vi "例10.7  保存单幅图像.vi"() -> ()   [LabVIEW 2017]
panel:
  out "Image Out":T1(plugin-control)
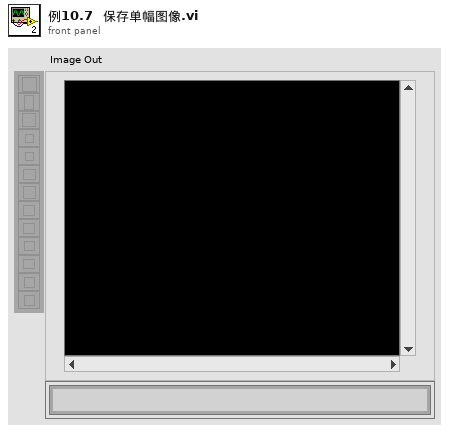
[diagram p1: front panel]
types:
  T1 = typedef "IMAQ Image.ctl" = refnum<image>
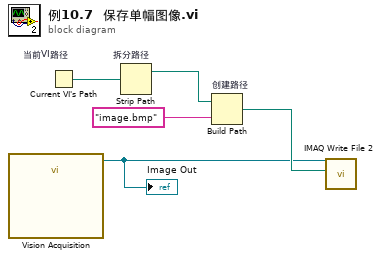
[diagram p0: block diagram]
diagram:
  n1 = call "Vision Acquisition"() -> ("Image Out"=w1:T1)  [unwired: 26 in, 1 out]
  "Image Out" <- w1
  n2 = Current VI's Path "当前VI路径"() -> (path=w4:path)
  n3 = Strip Path "拆分路径"(path=w4) -> (stripped path=w3:path)  [unwired: 1 out]
  n4 = Build Path "创建路径"(base path=w3, name or relative path="image.bmp") -> (appended path=w2:path)
  n5 = call-poly "IMAQ Write File 2"("File Path"=w2, "Image"=w1) -> ()  [unwired: 8 in, 2 out]
